vi "Last Ack Created Event.vi"(10 "Event":refnum<class "Event.lvclass">, 11 "jettl Msg Last Ack Created Event in":refnum<class "jettl Msg Last Ack Created Event.lvclass">) -> (3 "jettl Msg Last Ack Created Event out":refnum<class "jettl Msg Last Ack Created Event.lvclass">)   [LabVIEW 2021, in "jettl.lvlib" / "Last Ack Created Event Msg Strategy.lvlib" / "jettl Msg Last Ack Created Event.lvclass"]
uses:
  jettl Msg Last Ack Created Event.lvclass
  Event/Event.lvclass
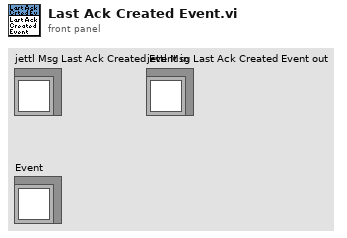
[diagram p1: front panel]
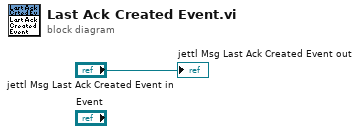
[diagram p0: block diagram]
diagram:
  "jettl Msg Last Ack Created Event out" <- "jettl Msg Last Ack Created Event in"
